vi "Get Trace Name.vi"(8 "error in (no error)":errorcluster {"code" format="%.0x"}, 9 "NameBufferSize (256)":i32=256, 10 "index":i32=1 caption="index (1)" format="%.0g", 11 "instrument handle":refnum<k15>) -> (0 "error out":errorcluster {"code" format="%.0x"}, 1 "name":string, 3 "instrument handle out":refnum<k15>)   [LabVIEW 2009, in "Keysight XSAn.lvlib"]
doc: "This VI returns the specific driver defined trace name that corresponds to the one-based index that the user specifies. If the value that the user passes for the Index parameter is less than one or greater than the value of the Trace Count property, the VI returns an empty string in the Name parameter and returns the Invalid Value error.\n\nSupported Models: All supported"
uses:
  <instrlib>/Keysight XSAn/Keysight XSAn.lvlib
  AgXSAn.dll
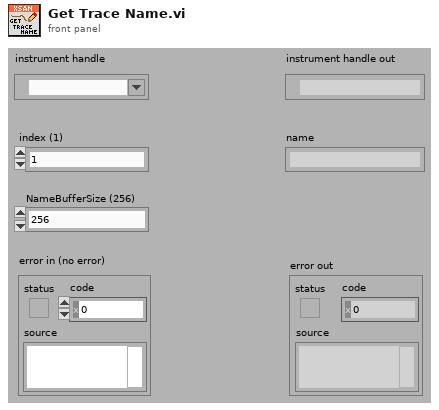
[diagram p1: front panel]
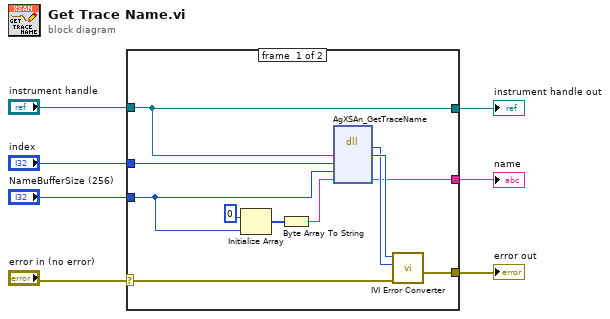
[diagram p0: block diagram]
diagram:
  n1 = case shown="No Error" "error in (no error)" {
    selector: "error in (no error)" -> [w13 w20]
    tunnel: [w14 w20] -> w6
    tunnel: "instrument handle" -> [w11 w19]
    tunnel: [w11 w19] -> w4
    tunnel: "index" -> [w10 _]
    tunnel: [w9 _] -> w2
    tunnel: "NameBufferSize (256)" -> [w8 _]
    frame #0 {
      n2 = Initialize Array(u8 0, w8) -> (w17:u8[])
      n3 = Byte Array To String(unsigned byte array=w17) -> (string=w16:string)
      n4 = dll-call lib="AgXSAn**.dll" fn="AgXSAn_GetTraceName" ("LabVIEW:IviSpecAn_GetTraceName")("instrument handle"=w11, "index"=w10, "name buffer size"=w8, "name"=w16) -> ("Status or Required Size"=w12:i32, "instrument handle"=w15:u32, "name"=w9:string)  [unwired: 5 in, 2 out]
      n5 = call <instrlib>:"IVI Error Converter.vi"("error in (no error)"=w13, "IVI error code (0)"=w12, "instrument handle"=w15) -> ("error out"=w14:errorcluster)  [unwired: 7 in, 1 out]
    }
    frame #1 {
    }
  }
  "error out" <- w6
  "instrument handle out" <- w4
  "name" <- w2
